vi "SetService.vi"(8 "error in":errorcluster, 10 "Properties":string[][](array[string]), 11 "Thing Info In":T2) -> (0 "error out":errorcluster, 3 "Thing Info Out":T2)   [LabVIEW 2015]
uses:
  <vilib>/httpClient/ClientHandle.ctl
  <vilib>/httpClient/POSTBuffer.vi
  <vilib>/httpClient/LabVIEWHTTPClient.lvlib
panel:
  out "final url":string
  out "reply body":string
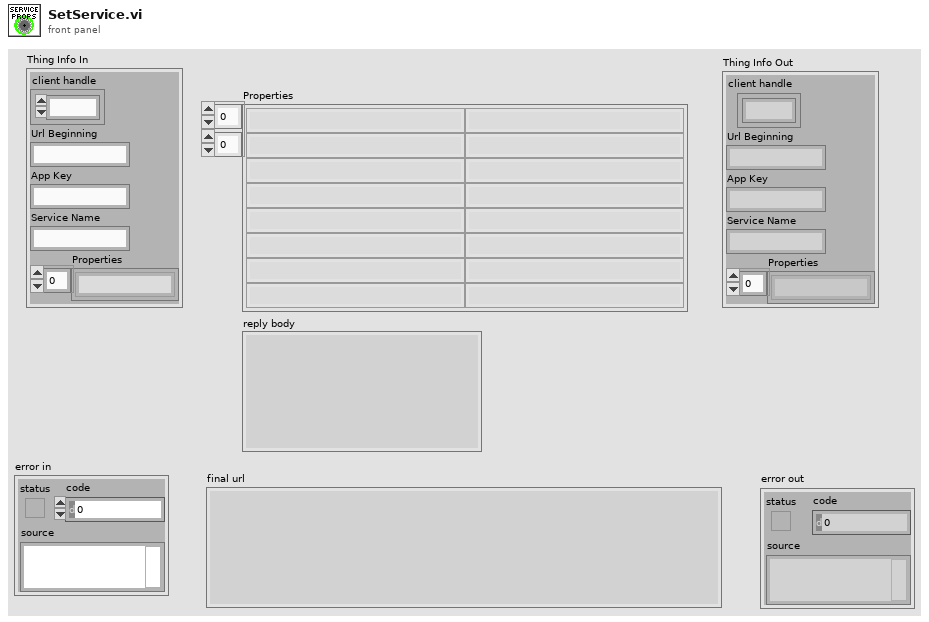
[diagram p1: front panel]
types:
  T1 = typedef "LabVIEWHTTPClient.lvlib/ClientHandle.ctl" = refnum<k1>
  T2 = cluster{"client handle":T1, "Url Beginning":string, "App Key":string, "Service Name":string, "Properties":string[]}
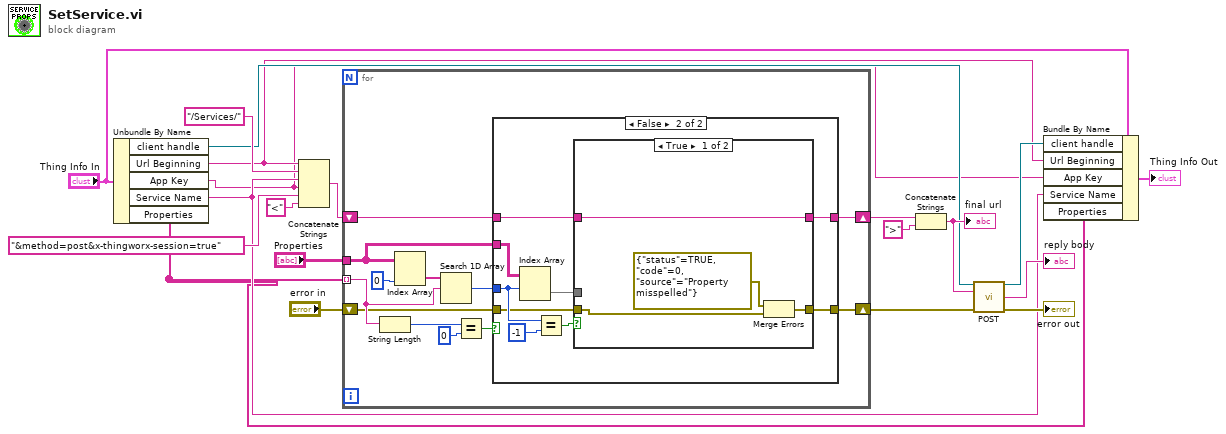
[diagram p0: block diagram]
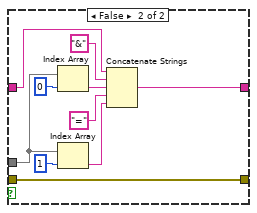
[diagram p3: hidden frame]
diagram:
  n1 = Unbundle By Name("Thing Info In") -> ("client handle"=w8:T1, "Url Beginning"=w6:string, "App Key"=w1:string, "Service Name"=w3:string, "Properties"=w2:string[])
  n2 = Concatenate Strings(w6, "/Services/" ("string"), w3, w1, "&method=post&x-thingworx-session=true" ("string"), "<" ("string")) -> (w15:string)
  n3 = for {
    tunnel: "Properties" -> [w30]
    shift-right: [w31] -> w14
    shift-left: w15 -> [w32]
    tunnel: w2 -> [w26] mode=indexing
    shift-right: [w21] -> w9
    shift-left: "error in" -> [w22]
    n4 = String Length(string=w26) -> (length=w25:i32)
    n5 = Index Array(array=w30, index (col)=0 ("disabled index (col)")) -> (element=w28:string[])  [unwired: 1 in]
    n6 = Search 1D Array(1D array=w28, element=w26) -> (index of element=w27:i32)  [unwired: 1 in]
    n7 = Equal?(x=w25, y=0) -> (x = y?=w23:bool)
    n8 = case shown="False" w23 {
      tunnel: w32 -> [w34 w43]
      tunnel: [w34 w42] -> w31
      tunnel: w30 -> [_ w40]
      tunnel: w27 -> [_ w39]
      tunnel: w22 -> [w33 w36]
      tunnel: [w33 w35] -> w21
      frame True {
      }
      frame False {
        n9 = Index Array(array=w40, index (row)=w39) -> (element=w38:string[])  [unwired: 1 in]
        n10 = Equal?(x=w39, y=-1) -> (x = y?=w37:bool)
        n11 = case shown="True" w37 {
          tunnel: w43 -> [w44 w56]
          tunnel: [w44 w54] -> w42
          tunnel: w38 -> [_ w53]
          tunnel: w36 -> [w47 w48]
          tunnel: [w45 w48] -> w35
          frame True {
            n12 = Merge Errors(errorcluster {"status"=TRUE, "code"=0, "source"="Property misspelled"} ("error in"), w47) -> (w45:errorcluster)
          }
          frame False {
            n13 = Index Array(array=w53, index=0) -> (element=w50:string)
            n14 = Index Array(array=w53, index=1) -> (element=w52:string)
            n15 = Concatenate Strings(w56, "&" ("string"), w50, "=" ("string"), w52) -> (w54:string)
          }
        }
      }
    }
  }
  n16 = Concatenate Strings(w14, ">" ("string")) -> (w13:string)
  "final url" <- w13
  n17 = call-poly <vilib>:"POST.vi"("client handle"=w8, "url"=w13, "error in (no error)"=w9) -> ("client handle out"=w7:T1, "body"=→"reply body":string, "error out"=→"error out":errorcluster)  [unwired: 9 in, 1 out]
  n18 = Bundle By Name(cluster="Thing Info In", "client handle"=w7, "Url Beginning"=w6, "App Key"=w1, "Service Name"=w3, "Properties"=w2) -> (→"Thing Info Out":T2)
